vi "test client.vi"() -> ()   [LabVIEW 2016]
uses:
  websocket client.lvclass
panel:
  out "error out":errorcluster
  in  "address":string="localhost"
  in  "port":u16=8095
  in  "url":string="dsfs"
  in  "error in":errorcluster
  in  "host header":string="sdfs"
  in  "subprotocols":string[](array[string])=["sdfs"]
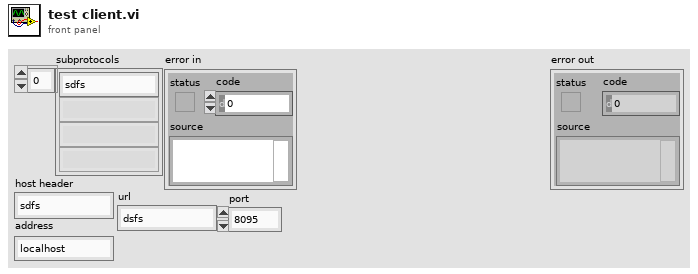
[diagram p1: front panel]
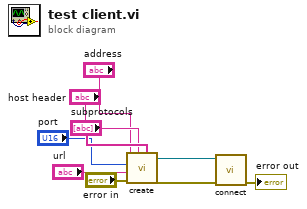
[diagram p0: block diagram]
diagram:
  n1 = call "create.vi"("subprotocols"="subprotocols", "host header"="host header", "error in"="error in", "url"="url", "port"="port", "address"="address") -> ("error out"=w8:errorcluster, "websocket client out"=w9:refnum<class "websocket client.lvclass">)  [unwired: 4 in]
  n2 = call "connect.vi"("error in"=w8, "websocket client in"=w9) -> ("error out"=→"error out":errorcluster)  [unwired: 8 in, 1 out]
